vi "RC_Client Client.vi"(8 "error in (no error)":errorcluster, 11 "RemoteControl in":refnum<class "RemoteControl.lvclass">) -> (0 "error out":errorcluster)   [LabVIEW 2019, in "RemoteControl.lvlib" / "RemoteControl.lvclass"]
uses:
  RemoteControl.lvclass
  8cfeec9d-4799-43e6-b258-77b28ef50c11.vi
panel:
  in  "milliseconds to wait":u32
  out "time (1 message) (ms)":u32
  out "messsages/s":dbl
  in  "remote port":u16=6341
  in  "address":string
  out "Parse Response":string
  out "Messages":i32
  in  "Stop":bool
  out "Command reponse":string
  out "Command":string
  out "commands":string[](array[string])
  # "CLIENT (API)"
  # "Connection info"
  # "Message Sent"
  # "Message Received"
  # "Metrics"
  # "client 1"
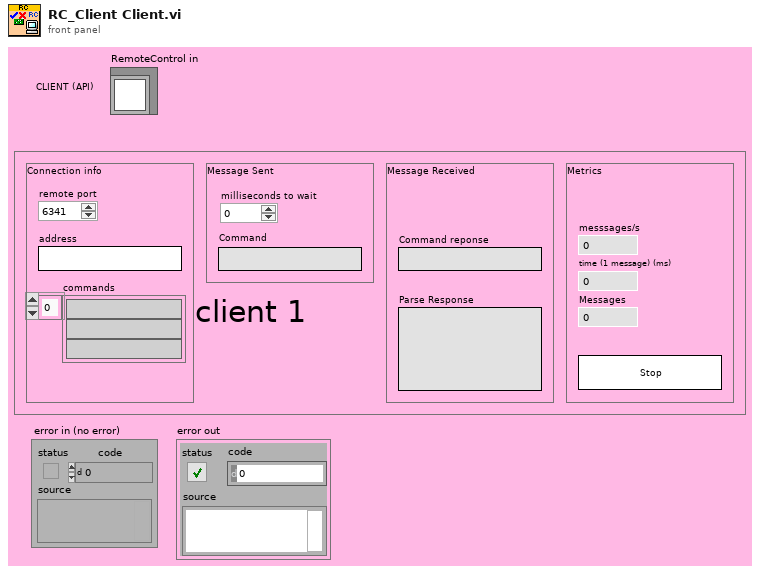
[diagram p1: front panel]
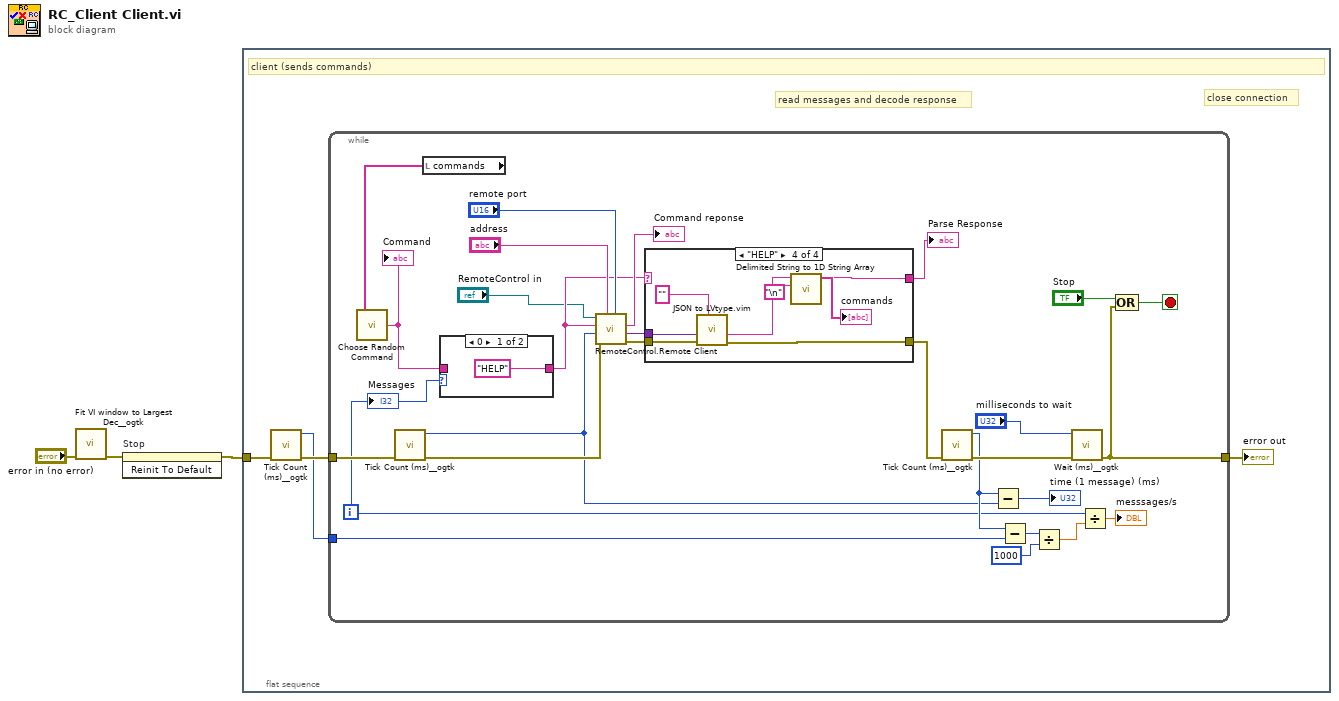
[diagram p0: block diagram]
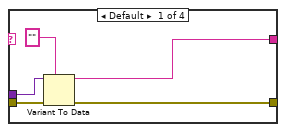
[diagram p3: hidden frame]
diagram:
  n1 = call <userlib>:"Fit VI window to Largest Dec__ogtk.vi"("error in (no error)"="error in (no error)") -> ("error out"=w3:errorcluster)  [unwired: 5 in, 1 out]
  n2 = invoke on="Stop" class="Bool" method="Reinit To Default"(error in=w3) -> (error out=w2:errorcluster)  [unwired: 2 in, 2 out]
  n3 = flat-sequence {
    tunnel: w2 -> [w4]
    frame #0 {
      # "close connection"
      # "read messages and decode response"
      # "client (sends commands)"
      n4 = call <userlib>:"Tick Count (ms)__ogtk.vi"("error in (no error)"=w4) -> ("error out"=w7:errorcluster, "millisecond timer value"=w6:u32)  [unwired: 9 in]
      n5 = while {
        tunnel: [w28] -> w5
        tunnel: w7 -> [w31]
        tunnel: w6 -> [w23]
        i -> [w16]
        stop <- w34 stop-if-true
        n6 = call <userlib>:"Tick Count (ms)__ogtk.vi"("error in (no error)"=w31) -> ("error out"=w20:errorcluster, "millisecond timer value"=w9:u32)  [unwired: 9 in]
        n7 = local read "commands"() -> (w13:string[])
        n8 = call "Choose Random Command.vi"("Array"=w13) -> ("String"=w12:string)
        "Command" <- w12
        n9 = case shown="0" w16 {
          tunnel: ["HELP" ("Command") w36] -> w10
          tunnel: w12 -> [_ w36]
          frame 0 {
          }
          frame Default {
          }
        }
        n10 = call "RemoteControl.Remote Client.vi"("Port"="remote port", "address"="address", "error in (no error)"=w20, "Data"=w9, "Command"=w10, "RemoteControl in"="RemoteControl in") -> ("error out"=w19:errorcluster, "Data out"=w21:variant, "Command out"=→"Command reponse":string)  [unwired: 2 in, 1 out]
        n11 = case shown="\"HELP\"" w10 {
          selector: w10 -> [_ w42 w44 _]
          tunnel: [w37 w42 w44 w47] -> w18
          tunnel: w21 -> [w41 _ _ w49]
          tunnel: [w38 w43 w45 w46] -> w17
          tunnel: w19 -> [w39 w43 w45 w50]
          frame Default {
            n12 = Variant To Data(error in=w39, type="", Variant=w41) -> (data=w37:string, error out=w38:errorcluster)
          }
          frame "open" {
          }
          frame "close" {
          }
          frame "HELP" {
            n13 = call "JSON to LVtype.vim"("type"="", "error in (no error)"=w50, "JSON Data in"=w49) -> ("error out"=w46:errorcluster, "Data out"=w47:string)  [unwired: 7 in]
            n14 = call <vilib>:"Delimited String to 1D String Array.vi"("delimiter"="\n", "delimited string"=w47) -> ("string array"=→"commands":string[])  [unwired: 9 in]
          }
        }
        "Parse Response" <- w18
        n15 = call <userlib>:"Tick Count (ms)__ogtk.vi"("error in (no error)"=w17) -> ("error out"=w30:errorcluster, "millisecond timer value"=w25:u32)  [unwired: 9 in]
        n16 = Subtract(x=w25, y=w9) -> (x-y=→"time (1 message) (ms)":u32)
        n17 = Subtract(x=w25, y=w23) -> (x-y=w24:u32)
        n18 = Divide(x=w24, y=u32 1000) -> (x/y=w33:dbl)
        n19 = call <userlib>:"Wait (ms)__ogtk.vi"("error in (no error)"=w30, "milliseconds to wait"="milliseconds to wait") -> ("error out"=w28:errorcluster)  [unwired: 8 in, 1 out]
        n20 = Divide(x=w16, y=w33) -> (x/y=→"messsages/s":dbl)
        n21 = Compound Arithmetic op=OR("Stop", w28) -> (w34:bool)
        "Messages" <- w16
      }
      "error out" <- w5
    }
  }
